vi "Autofit Worksheet.vi"(5 "Start Cell":string="A1", 7 "End Cell":string="Z1000", 8 "error in (no error)":errorcluster, 11 "Report In":refnum<class "NI_report.lvclass">) -> (0 "error out":errorcluster, 3 "Report Out":refnum<class "NI_report.lvclass">)   [LabVIEW 2014]
uses:
  <vilib>/Utility/NIReport.llb/NI_report.lvclass
  <vilib>/Utility/NIReport.llb/Excel/NI_Excel.lvclass
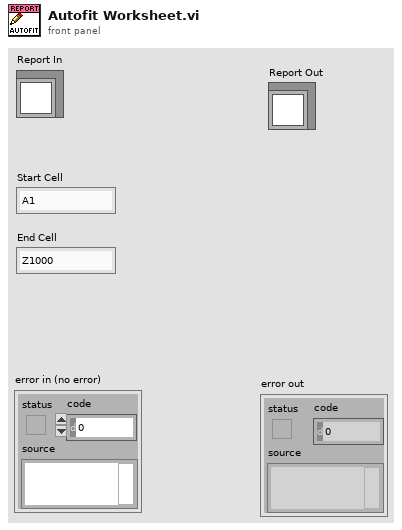
[diagram p1: front panel]
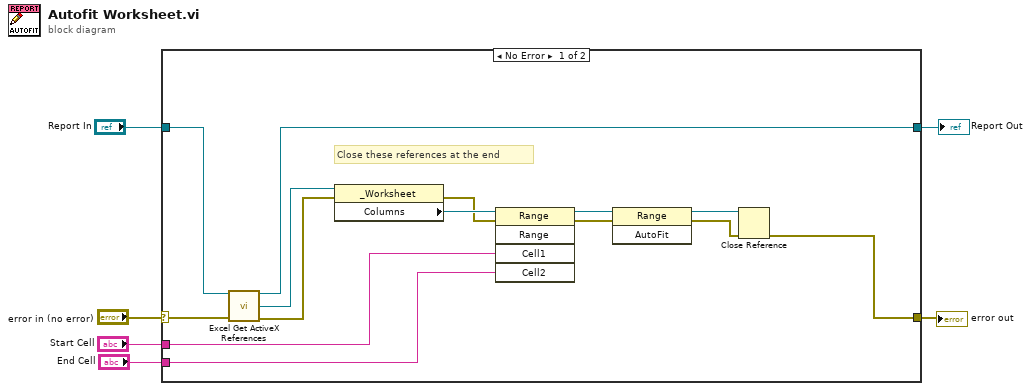
[diagram p0: block diagram]
diagram:
  n1 = case shown="No Error" "error in (no error)" {
    selector: "error in (no error)" -> [w20 w22]
    tunnel: [w7 w22] -> w6
    tunnel: "Report In" -> [w16 w21]
    tunnel: [w15 w21] -> w3
    tunnel: "Start Cell" -> [w10 _]
    tunnel: "End Cell" -> [w9 _]
    frame No Error {
      # "Close these references at the end"
      n2 = call <vilib>:"Excel Get ActiveX References.vi"("report in"=w16, "error in (no error)"=w20) -> ("report out"=w15:refnum<class "NI_report.lvclass">, "Excel._Worksheet"=w8:refnum<k7>, "error out"=w17:errorcluster)  [unwired: 7 in, 4 out]
      n3 = property class="_Worksheet"(reference=w8, error in=w17) -> (error out=w11:errorcluster, "Columns"=w14:refnum<k7>)  [unwired: 1 out]
      n4 = invoke class="Range" method="Range"(reference=w14, error in=w11, "Cell1"=w10, "Cell2"=w9) -> (reference out=w13:refnum<k7>, error out=w12:errorcluster)  [unwired: 1 in, 3 out]
      n5 = invoke class="Range" method="AutoFit"(reference=w13, error in=w12) -> (reference out=w18:refnum<k7>, error out=w19:errorcluster)  [unwired: 1 in, 1 out]
      n6 = Close Reference(reference=w18, error in (no error)=w19) -> (error out=w7:errorcluster)
    }
    frame Error {
    }
  }
  "error out" <- w6
  "Report Out" <- w3
